vi "Wait for Exit.vi"(6 "deadline":T1={"mode"=enum."Relative", "deadline (ms)"=30000}, 8 "error in (no error)":errorcluster, 11 "subprocess in":refnum<class "Subprocess.lvclass">) -> (0 "error out":errorcluster, 2 "return code":u8, 3 "subprocess out":refnum<class "Subprocess.lvclass">)   [LabVIEW 2020, in "NI_Subprocess.lvlib" / "Subprocess.lvclass"]
doc: "Wait for the subprocess to exit, and record its return code."
uses:
  <vilib>/Subprocess/Subprocess/Subprocess.lvclass
  <vilib>/Utility/Deadline/Deadline.ctl
  <vilib>/Utility/Deadline/Mode.ctl
  <vilib>/Subprocess/Subprocess/Subprocess.lvclass/Subprocess.ctl
  lviosrg.dll
  <vilib>/Utility/error.llb/Error Cluster From Error Code.vi
  <vilib>/ErrorRing/Error Ring.xnode
  <vilib>/Utility/Deadline/NI_Deadline.lvlib
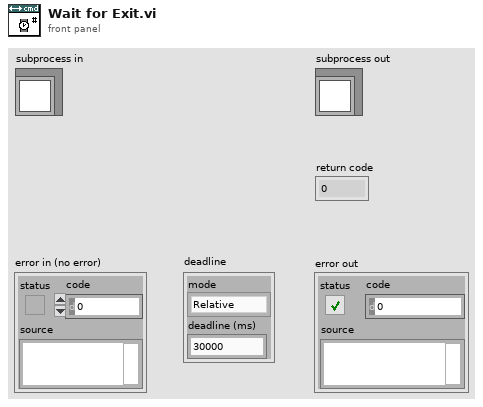
[diagram p1: front panel]
types:
  T1 = typedef "NI_Deadline.lvlib/Deadline.ctl" = cluster{"mode":T2, "deadline (ms)":u32}
  T2 = typedef "NI_Deadline.lvlib/Mode.ctl" = enum16{"Relative", "Use deadline", "Wait forever", "Nonblocking", "N/A"}
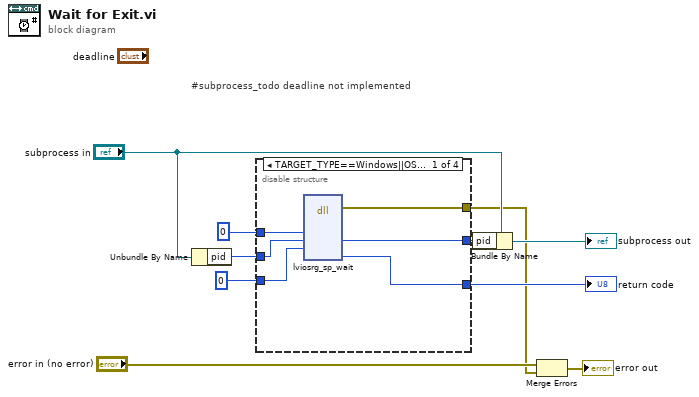
[diagram p0: block diagram]
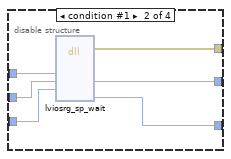
[diagram p2: hidden frame]
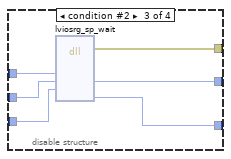
[diagram p3: hidden frame]
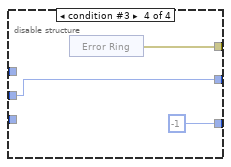
[diagram p4: hidden frame]
diagram:
  # "#subprocess_todo deadline not implemented"
  n1 = Unbundle By Name("subprocess in") -> ("pid"=w7:u64)
  n2 = disable-structure shown="TARGET_TYPE==Windows||OS==Win" {
    disable-tunnel: w7 -> [w15 w21 w27 w30]
    disable-tunnel: [w16 w22 w28 -1 ("exitCode")] -> w8
    disable-tunnel: [w14 w20 w26 w30] -> w6
    disable-tunnel: u8 0 ("block") -> [w13 w18 w24 _]
    disable-tunnel: 0 ("errno") -> [w12 w19 w25 _]
    disable-tunnel: [w11 w17 w23 w29] -> w2
    frame condition #0 (active) {
      n3 = dll-call lib="lviosrg.dll" fn="lviosrg_sp_wait"("errno"=w12, "process"=w15, "block"=w13) -> (error out=w11:errorcluster, "process"=w14:u64, "exitCode"=w16:i32)  [unwired: 9 in, 1 out]
    }
    frame condition #1 {
      n4 = dll-call lib="lviosrg.*" fn="lviosrg_sp_wait"("errno"=w19, "process"=w21, "block"=w18) -> (error out=w17:errorcluster, "process"=w20:u64, "exitCode"=w22:i32)  [unwired: 9 in, 1 out]
    }
    frame condition #2 {
      n5 = dll-call lib="lviosrg.*" fn="lviosrg_sp_wait"("errno"=w25, "process"=w27, "block"=w24) -> (error out=w23:errorcluster, "process"=w26:u64, "exitCode"=w28:i32)  [unwired: 9 in, 1 out]
    }
    frame condition #3 {
      n6 = xnode "Error Ring"() -> ("error out"=w29:errorcluster)
    }
  }
  "return code" <- w8
  n7 = Bundle By Name(cluster="subprocess in", "pid"=w6) -> (→"subprocess out":refnum<class "Subprocess.lvclass">)
  n8 = Merge Errors("error in (no error)", w2) -> (→"error out":errorcluster)
